vi "Create_pos_for_all_ch.vi"() -> (1 "Positions for all Ch":T1(array[cluster]) {"Z" format="%.2f"; "Y" format="%.2f"; "X" format="%.2f"})   [LabVIEW 2010]
uses:
  Globals/Meas_global.vi
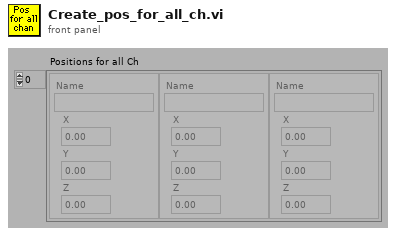
[diagram p1: front panel]
types:
  T1 = cluster{"Name":string, "X":dbl, "Y":dbl, "Z":dbl}[]
  T2 = typedef "Analysis_info_cluster.ctl" = cluster{"Colour":u32, "Inst type":T3, "Inst name":string, "Symbol":string, "Code name":string, "Extra Info":string, "Inst Array":T4, "Index":i32, "Voltage Index":i32, "Extra Titles":string[], "Extra Values":string[]}
  T3 = typedef "Inst_type.ctl" = enum16{"Propeller anemometer", "Raw voltage", "Pressure Transducer", "Pitot-static tube", "Preston tube", "Hot wire", "Cross wire 1", "Cross wire 2", "Generic Linear", "Generic Polynomial", "Generic BackPoly", "Fast FID", "Thermocouple", "Cold wire", "Pulsed Wire", "LDA Vel", "LDA Tran time", "LDA Arr time"}
  T4 = typedef "Instrument_Array.ctl" = enum16{"PWA", "LDA", "Analogue"}
  T5 = typedef "Analysis_type_cluster.ctl" = cluster{"Analysis type":T6, "Indicies":i32[], "Name":string, "Inst Array":T4, "Info index":i32}
  T6 = typedef "Analysis_type_Enum.ctl" = enum16{"Slow Response", "Fast Response", "Weighted Fast Response", "Fast FID", "Weighted Fast FID", "Cross Wire", "Weighted Cross Wire", "Weighted LDA"}
  T7 = cluster{"Name":string, "X":dbl, "Y":dbl, "Z":dbl}
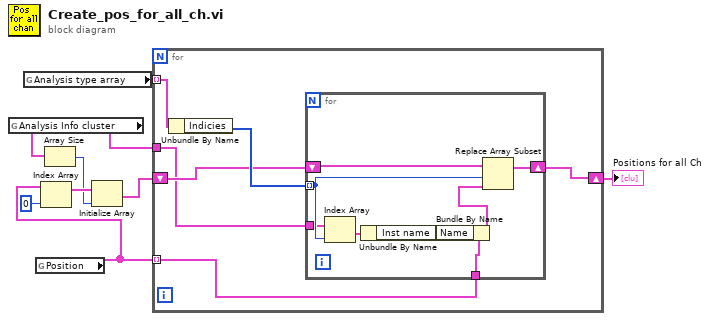
[diagram p0: block diagram]
diagram:
  n1 = global read "Meas_global.vi" "Analysis Info cluster"() -> (w2:T2[])
  n2 = global read "Meas_global.vi" "Analysis type array"() -> (w8:T5[])
  n3 = global read "Meas_global.vi" "Position"() -> (w5:T1)
  n4 = Index Array(array=w5, index=0) -> (element=w4:T7)
  n5 = Array Size(array=w2) -> (size(s)=w3:i32)
  n6 = Initialize Array(w4, w3) -> (w7:T1)
  n7 = for {
    tunnel: w5 -> [w10] mode=indexing
    tunnel: w8 -> [w14] mode=indexing
    shift-right: [w11] -> w1
    shift-left: w7 -> [w12]
    tunnel: w2 -> [w9]
    n8 = Unbundle By Name(w14) -> ("Indicies"=w13:i32[])
    n9 = for {
      shift-right: [w21] -> w11
      shift-left: w12 -> [w22]
      tunnel: w13 -> [w19] mode=indexing
      tunnel: w10 -> [w20]
      tunnel: w9 -> [w18]
      n10 = Index Array(array=w18, index=w19) -> (element=w17:T2)
      n11 = Unbundle By Name(w17) -> ("Inst name"=w16:string)
      n12 = Bundle By Name(cluster=w20, "Name"=w16) -> (w15:T7)
      n13 = Replace Array Subset(array=w22, new element=w15, index=w19) -> (w21:T1)
    }
  }
  "Positions for all Ch" <- w1
